vi "Generate output.vi"(6 "index":i32, 7 "new treatment":bool, 8 "error in":errorcluster, 9 "Current treatment":T1, 10 "Data in":T2, 11 "Run info":T3) -> (0 "error out":errorcluster, 1 "Current treatment out":T1, 2 "Data out":T2, 3 "Run info out":T3)   [LabVIEW 2012]
uses:
  Run info.ctl
  Data.ctl
  Treatment.ctl
  <vilib>/Analysis/NI_AALBase.lvlib
  <vilib>/Analysis/NI_AALPro.lvlib
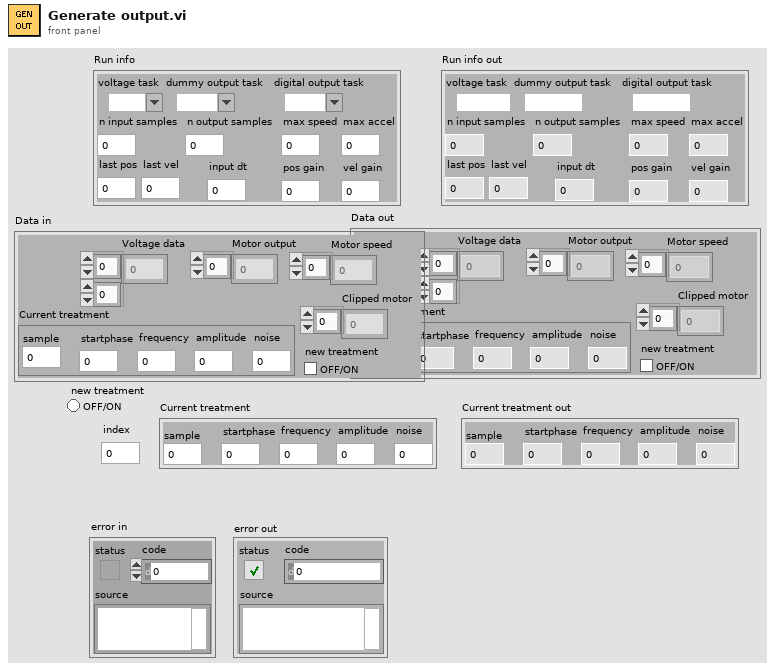
[diagram p1: front panel]
types:
  T1 = typedef "Treatment.ctl" = cluster{"sample":dbl, "startphase":dbl, "frequency":dbl, "amplitude":dbl, "noise":dbl}
  T2 = typedef "Data.ctl" = cluster{"Voltage data":dbl[][], "Motor output":dbl[], "Current treatment":T1, "Motor speed":dbl[], "Clipped motor":dbl[], "new treatment":bool}
  T3 = typedef "Run info.ctl" = cluster{"voltage task":refnum<k21>, "dummy output task":refnum<k21>, "digital output task":refnum<k21>, "n input samples":i32, "n output samples":i32, "max speed":dbl, "max accel":dbl, "last pos":dbl, "last vel":dbl, "pos gain":dbl, "vel gain":dbl, "input dt":dbl}
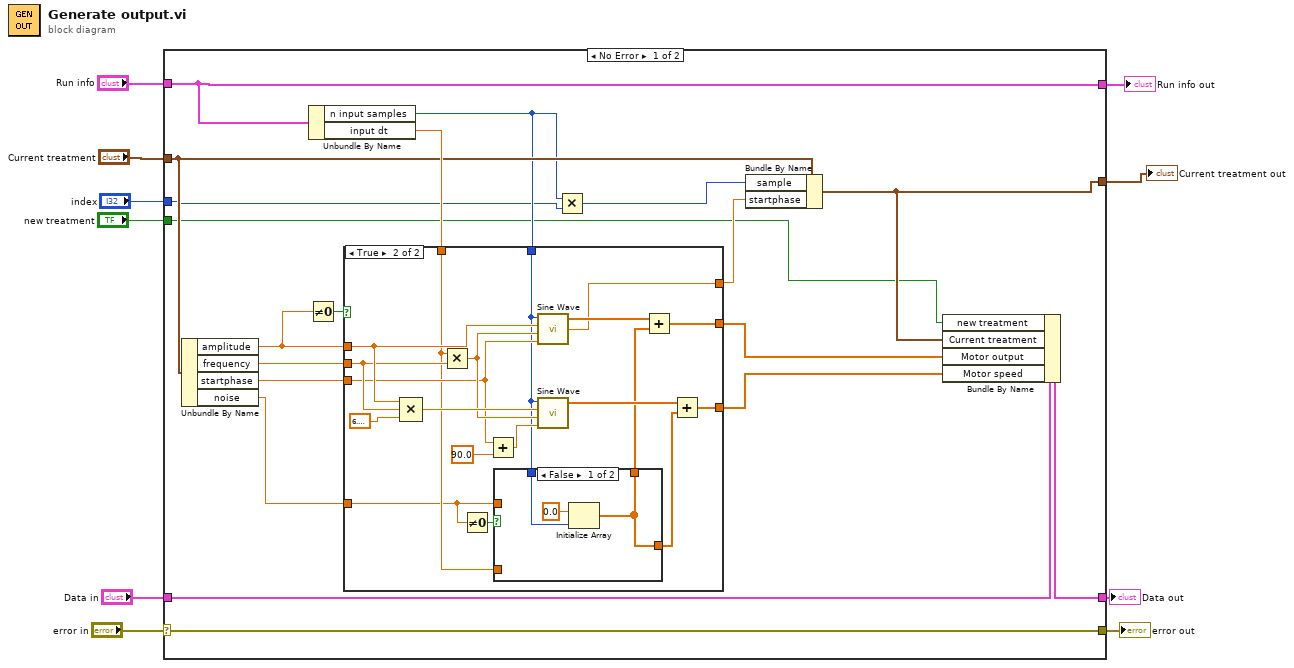
[diagram p0: block diagram]
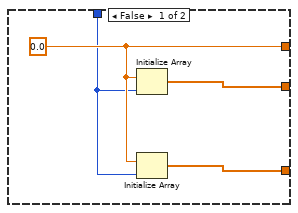
[diagram p2: hidden frame]
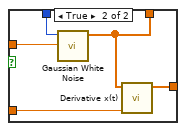
[diagram p3: hidden frame]
diagram:
  n1 = case shown="No Error" "error in" {
    selector: "error in" -> [w26 w63]
    tunnel: "Run info" -> [w29 w64]
    tunnel: [w26 w63] -> w8
    tunnel: [w29 w64] -> w7
    tunnel: "Current treatment" -> [w19 w61]
    tunnel: "Data in" -> [w28 w62]
    tunnel: [w27 w62] -> w5
    tunnel: [w12 w61] -> w3
    tunnel: "new treatment" -> [w11 _]
    tunnel: "index" -> [w15 _]
    frame No Error {
      n2 = Unbundle By Name(w19) -> ("amplitude"=w20:dbl, "frequency"=w25:dbl, "startphase"=w17:dbl, "noise"=w13:dbl)
      n3 = Not Equal To 0?(x=w20) -> (x != 0?=w21:bool)
      n4 = Unbundle By Name(w29) -> ("n input samples"=w16:i32, "input dt"=w23:dbl)
      n5 = case shown="True" w21 {
        tunnel: w16 -> [w30 w41]
        tunnel: w20 -> [_ w52]
        tunnel: w25 -> [_ w49]
        tunnel: [w32 w35] -> w24
        tunnel: w23 -> [_ w40]
        tunnel: [w33 w37] -> w22
        tunnel: [w31 w43] -> w18
        tunnel: w17 -> [_ w42]
        tunnel: w13 -> [_ w38]
        frame False {
          w31 = 0.0
          n6 = Initialize Array(w31, w30) -> (w33:dbl[])
          n7 = Initialize Array(w31, w30) -> (w32:dbl[])
        }
        frame True {
          n8 = Compound Arithmetic op=MULTIPLY(w52, w49, 6.283185307179586) -> (w50:dbl)
          n9 = Multiply(x=w40, y=w49) -> (x*y=w47:dbl)
          n10 = Not Equal To 0?(x=w38) -> (x != 0?=w39:bool)
          n11 = Add(x=w42, y=90.0) -> (x+y=w45:dbl)
          n12 = case shown="False" w39 {
            tunnel: w38 -> [_ w60]
            tunnel: w41 -> [w55 w59]
            tunnel: w40 -> [_ w58]
            tunnel: [w53 w57] -> w36
            tunnel: [w53 w56] -> w34
            frame False {
              n13 = Initialize Array(0.0 ("element"), w55) -> (w53:dbl[])
            }
            frame True {
              n14 = call <vilib>:"Gaussian White Noise.vi"("standard deviation"=w60, "samples"=w59) -> ("Gaussian noise pattern"=w57:dbl[])  [unwired: 8 in, 1 out]
              n15 = call <vilib>:"Derivative x(t).vi"("dt"=w58, "X"=w57) -> ("dX/dt"=w56:dbl[])  [unwired: 8 in, 1 out]
            }
          }
          n16 = call <vilib>:"Sine Wave.vi"("samples"=w41, "amplitude"=w52, "frequency"=w47, "phase in"=w42) -> ("sine wave"=w46:dbl[], "phase out"=w43:dbl)  [unwired: 1 in, 1 out]
          n17 = call <vilib>:"Sine Wave.vi"("samples"=w41, "amplitude"=w50, "frequency"=w47, "phase in"=w45) -> ("sine wave"=w48:dbl[])  [unwired: 1 in, 2 out]
          n18 = Add(x=w46, y=w36) -> (x+y=w37:dbl[])
          n19 = Add(x=w48, y=w34) -> (x+y=w35:dbl[])
        }
      }
      n20 = Multiply(x=w16, y=w15) -> (x*y=w14:i32)
      n21 = Bundle By Name(cluster=w19, "sample"=w14, "startphase"=w18) -> (w12:T1)
      n22 = Bundle By Name(cluster=w28, "new treatment"=w11, "Current treatment"=w12, "Motor output"=w22, "Motor speed"=w24) -> (w27:T2)
    }
    frame Error {
    }
  }
  "Data out" <- w5
  "Run info out" <- w7
  "error out" <- w8
  "Current treatment out" <- w3
